vi "string2num.vi"(2 "string 2":string) -> (7 "Result":dbl)   [LabVIEW 2013]
uses:
  <vilib>/express/express arith-compare/Formula/XNode/ExpressFormulaBlockNode.xnode
panel:
  out "error out":errorcluster
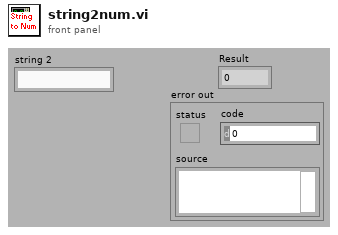
[diagram p1: front panel]
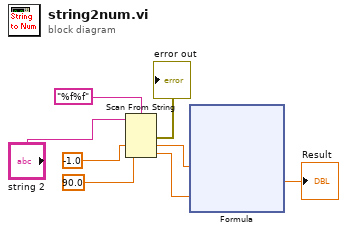
[diagram p0: block diagram]
diagram:
  n1 = Scan From String(format string="%f%f", input string="string 2", default 1=-1.0 ("default value 1"), default 2=90.0 ("default value 2")) -> (error out=→"error out":errorcluster, output 1=w4:dbl, output 2=w3:dbl)  [unwired: 2 in, 2 out]
  n2 = xnode "Formula"("factor"=w4, "exp"=w3) -> ("Result"=→"Result":dbl)  [unwired: 1 in, 1 out]
